vi "PH_PSDBWriter.read DB.vi"(2 "error in":errorcluster, 3 "Instance Name":string) -> (0 "error out":errorcluster, 1 "PSDB Subsystem":string)   [LabVIEW 2014, in "PH_PSDBWriter.lvlib"]
doc: "This VI reads certain data base entries of the instance \"PHELIX_PSDB-Writer\"."
uses:
  PH_PSDBWriter.lvlib
  PH_Common/PH_Common.lvlib
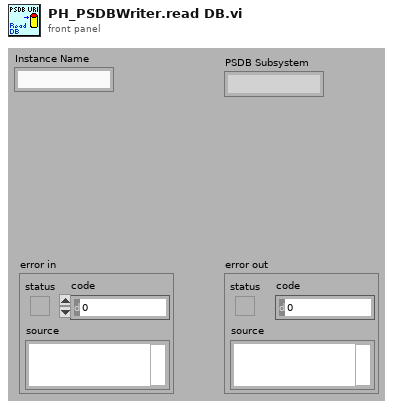
[diagram p1: front panel]
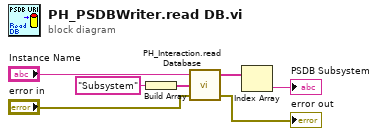
[diagram p0: block diagram]
diagram:
  n1 = Build Array("Subsystem" ("element")) -> (w3:string[])
  n2 = call "PH_Interaction.read Database.vi"("error in (no error)"="error in", "Strings to search for"=w3, "DB Entry to read"="Instance Name") -> ("error out"=→"error out":errorcluster, "Values"=w2:string[])  [unwired: 1 in]
  n3 = Index Array(array=w2) -> (element=→"PSDB Subsystem":string)  [unwired: 1 in]
